vi "Base64_Encode CORE.vi"(1 "base64 set":u8[](array[numeric]), 2 "String":string) -> (0 "string":string)   [LabVIEW 2013, in "Serializer.Base64.lvclass"]
doc: "20250509 - CORE function created to allow charset variable input for fast Base64url encoding"
uses:
  Serializer.Base64.lvclass
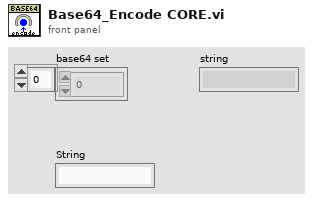
[diagram p1: front panel]
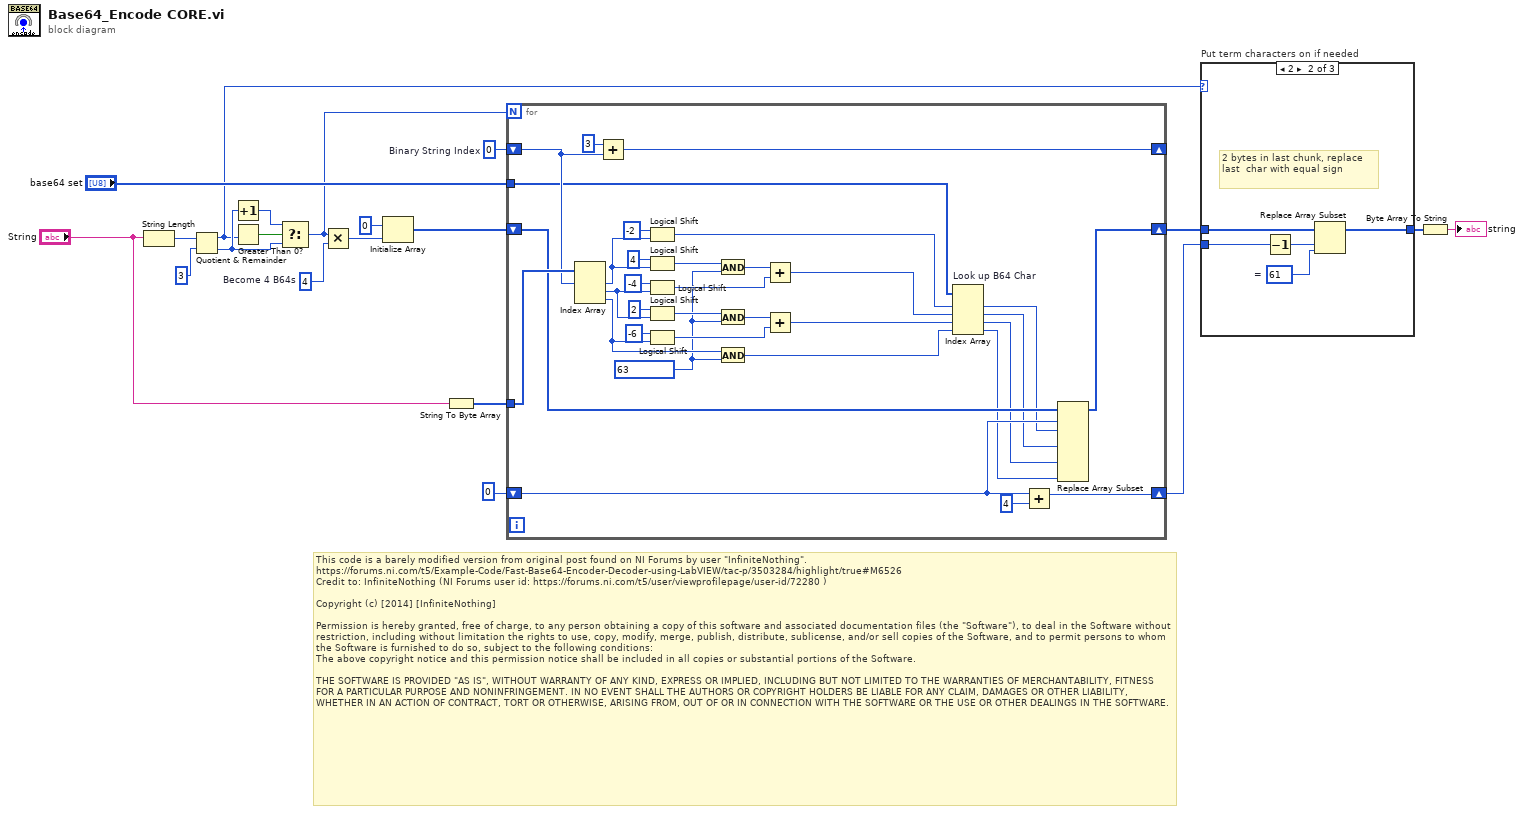
[diagram p0: block diagram]
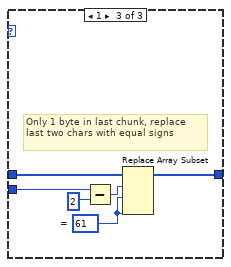
[diagram p3: hidden frame]
diagram:
  w13 = 4  # Become 4 B64s
  w9 = 0  # Binary String Index
  # "This code is a barely modified version from original post found on NI Forums by user \"InfiniteNothing\".\nhttps://forums.ni.com/t5/Example-Code/Fast-Base64-Encoder-Decoder-using-LabVIEW/tac-p/3503284/highlight/true#M6526\nCredit to: InfiniteNothing (NI Forums user id: https://forums.ni.com/t5/user/viewprofilepage/user-id/72280 )\n\nCopyright (c) [2014] [InfiniteNothing]\n\nPermission is hereby granted, free of charge, to any person obtaining a copy of this software and associated documentation files (the \"Software\"), to deal in the Software without restriction, including without limitation the rights to use, copy, modify, merge, publish, distribute, sublicense, and/or sell copies of the Software, and to permit persons to whom the Software is furnished to do so, subject to the following conditions:\nThe above copyright notice and this permission notice shall be included in all copies or substantial portions of the Software.\n\nTHE SOFTWARE IS PROVIDED \"AS IS\", WITHOUT WARRANTY OF ANY KIND, EXPRESS OR IMPLIED, INCLUDING BUT NOT LIMITED TO THE WARRANTIES OF MERCHANTABILITY, FITNESS FOR A PARTICULAR PURPOSE AND NONINFRINGEMENT. IN NO EVENT SHALL THE AUTHORS OR COPYRIGHT HOLDERS BE LIABLE FOR ANY CLAIM, DAMAGES OR OTHER LIABILITY, WHETHER IN AN ACTION OF CONTRACT, TORT OR OTHERWISE, ARISING FROM, OUT OF OR IN CONNECTION WITH THE SOFTWARE OR THE USE OR OTHER DEALINGS IN THE SOFTWARE."
  n1 = String Length(string="String") -> (length=w2:i32)
  n2 = Quotient & Remainder(x=w2, y=3 ("Chunks of 3 U8s")) -> (x-y*floor(x/y)=w4:i32, floor(x/y)=w6:i32)
  n3 = Increment(x=w6) -> (x+1=w7:i32)
  n4 = Greater Than 0?(x=w4) -> (x > 0?=w5:bool)
  n5 = Select(t=w7, s=w5, f=w6) -> (s? t:f=w11:i32)
  n6 = Multiply(x=w11, y=w13) -> (x*y=w12:i32)
  n7 = Initialize Array(u8 0 ("element"), w12) -> (w15:u8[])
  n8 = String To Byte Array(string="String") -> (unsigned byte array=w16:u8[])
  n9 = for {
    N: w11 -> [_]
    tunnel: w16 -> [w53]
    shift-right: [w51] -> _
    shift-left: w9 -> [w52]
    shift-right: [w48] -> w1
    shift-left: 0 ("B64 String Index") -> [w34]
    shift-right: [w35] -> w17
    shift-left: w15 -> [w36]
    tunnel: "base64 set" -> [w21]
    w22 = u8 63 ("y")
    n10 = Index Array(array=w53, index #1=w52) -> (element #1=w46:u8, element #2=w41:u8, element #3=w38:u8)  [unwired: 2 in]
    n11 = Add(x=3 ("Chunks of 3 U8s"), y=w52) -> (x+y=w51:i32)
    n12 = Logical Shift(y=i8 -2, x=w46) -> (x << y=w47:u8)
    n13 = Logical Shift(y=i8 4, x=w46) -> (x << y=w29:u8)
    n14 = Logical Shift(y=i8 -4, x=w41) -> (x << y=w43:u8)
    n15 = Logical Shift(y=i8 2, x=w41) -> (x << y=w26:u8)
    n16 = Logical Shift(y=i8 -6, x=w38) -> (x << y=w39:u8)
    n17 = And(x=w29, y=w22) -> (x .and. y?=w28:u8)
    n18 = And(x=w26, y=w22) -> (x .and. y?=w25:u8)
    n19 = And(x=w38, y=w22) -> (x .and. y?=w37:u8)
    n20 = Add(x=w28, y=w43) -> (x+y=w27:u8)
    n21 = Add(x=w25, y=w39) -> (x+y=w24:u8)
    n22 = Index Array "Look up B64 Char"(array=w21, index #1=w47, index #2=w27, index #3=w24, index #4=w37) -> (element #1=w33:u8, element #2=w32:u8, element #3=w31:u8, element #4=w30:u8)
    n23 = Add(x=w34, y=4 ("Become 4 B64s")) -> (x+y=w48:i32)
    n24 = Replace Array Subset(array=w36, new element #1=w33, index #1=w34, new element #2=w32, new element #3=w31, new element #4=w30) -> (w35:u8[])  [unwired: 3 in]
  }
  n25 = case "Put term characters on if needed" shown="2" w4 {
    tunnel: w17 -> [w54 w59 w65]
    tunnel: [w54 w58 w64] -> w3
    tunnel: w1 -> [_ w57 w62]
    frame 0, Default {
      # "All chunks had 3 bytes. Do nothing"
    }
    frame 2 {
      w55 = u8 61  # =
      # "2 bytes in last chunk, replace last  char with equal sign"
      n26 = Decrement(x=w57) -> (x-1=w56:i32)
      n27 = Replace Array Subset(array=w59, new element=w55, index=w56) -> (w58:u8[])
    }
    frame 1 {
      w60 = u8 61  # =
      # "Only 1 byte in last chunk, replace last two chars with equal signs"
      n28 = Subtract(x=w62, y=2) -> (x-y=w63:i32)
      n29 = Replace Array Subset(array=w65, new element #1=w60, index #1=w63, new element #2=w60) -> (w64:u8[])  [unwired: 1 in]
    }
  }
  n30 = Byte Array To String(unsigned byte array=w3) -> (string=→"string":string)
